vi "Cálculo_Velocidade_Líquidos.vi"(6 "Diâmetro Tubulação [m]":dbl, 9 "SKM-FI-WF":dbl, 10 "SKM-AI-KF_COR":dbl, 11 "SKM-FIC-KF_COR":dbl) -> (1 "Velocidade Líquido [m/s]":dbl, 2 "Velocidade Água [m/s]":dbl, 3 "Velocidade Querosene [m/s]":dbl)   [LabVIEW 2019]
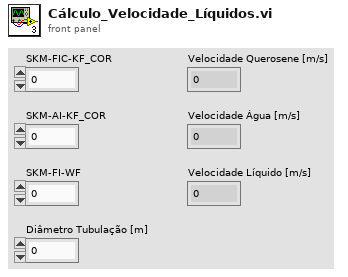
[diagram p1: front panel]
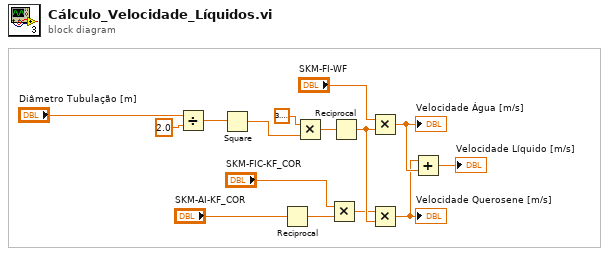
[diagram p0: block diagram]
diagram:
  n1 = Divide(x="Diâmetro Tubulação [m]", y=2.0) -> (x/y=w8:dbl)
  n2 = Square(x=w8) -> (x^2=w5:dbl)
  n3 = Reciprocal(x="SKM-AI-KF_COR") -> (1/x=w2:dbl)
  n4 = Multiply(x=3.141592653589793, y=w5) -> (x*y=w9:dbl)
  n5 = Multiply(x="SKM-FIC-KF_COR", y=w2) -> (x*y=w10:dbl)
  n6 = Reciprocal(x=w9) -> (1/x=w12:dbl)
  n7 = Multiply(x="SKM-FI-WF", y=w12) -> (x*y=w14:dbl)
  "Velocidade Água [m/s]" <- w14
  n8 = Multiply(x=w10, y=w12) -> (x*y=w13:dbl)
  "Velocidade Querosene [m/s]" <- w13
  n9 = Add(x=w13, y=w14) -> (x+y=→"Velocidade Líquido [m/s]":dbl)
